vi "getValueSimple.vi"() -> ()   [LabVIEW 2018]
panel:
  in  "input":dbl
  out "value":dbl
  out "error out":errorcluster
  in  "error in (no error)":errorcluster
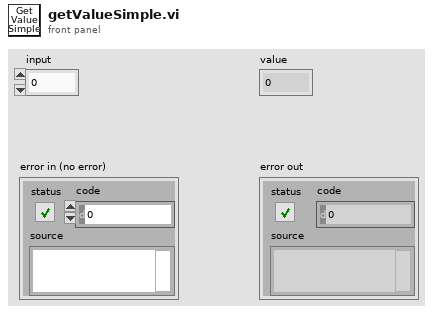
[diagram p1: front panel]
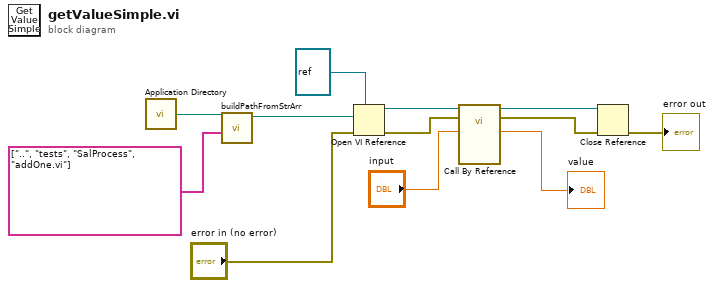
[diagram p0: block diagram]
diagram:
  n1 = call <vilib>:"Application Directory.vi"() -> ("Application Directory"=w12:path)
  n2 = call "buildPathFromStrArr.vi"("String Array"=string[] ["..", "tests", "SalProcess", "addOne.vi"], "Root Path"=w12) -> ("Absolute Path"=w10:path)  [unwired: 9 in]
  n3 = Open VI Reference(type specifier VI Refnum (for type only)=refnum<vi> refnum, vi path=w10, error in (no error)="error in (no error)") -> (vi reference=w7:refnum<vi>, error out=w6:errorcluster)  [unwired: 3 in]
  n4 = call-by-ref "?"(reference=w7, error in=w6, "input"="input") -> (reference out=w4:refnum<vi>, error out=w3:errorcluster, "value"=→"value":dbl)  [unwired: 9 in, 1 out]
  n5 = Close Reference(reference=w4, error in (no error)=w3) -> (error out=→"error out":errorcluster)
